vi "Main_spb.vi"() -> ()   [LabVIEW 2018]
uses:
  <vilib>/Platform/TimedLoop/XDataNode/timing_clust.ctl
  <vilib>/Platform/TimedLoop/XDataNode/nitl_modes.ctl
  <vilib>/Platform/TimedLoop/XDataNode/wakeup.ctl
  <vilib>/rvi/eio/common/nirviEmuTemplateMethod_errors.vi
  <vilib>/rvi/Emulation/niFpgaGetClockAttributes.vi
  <vilib>/rvi/Emulation/niFpgaSctlEmulationGetInTimedLoop.vi
  <vilib>/rvi/Emulation/niFpgaEmulationReportErrorSimple.vi
  <vilib>/rvi/Emulation/niFpgaProcessEmulError.vi
  <vilib>/rvi/Emulation/niFpgaCriticalErrorInLSC.vi
  <vilib>/rvi/DataTransferAndStorage/Container/Common/niFpgaContainerGetUniqueNameForEmu.vi
  <vilib>/rvi/Memory/Memory_Emulation/niFpgaMemoryFastEmulationDramWriteAndRequestData.vi
  <vilib>/rvi/Memory/Memory_Emulation/niFpgaMemoryEmulationDramWriteAndRequestData.vi
  <vilib>/rvi/Memory/Memory_Emulation/niFpgaMemoryEmulationDramWriteAndRequestDataApplyByteEnables.vi
  <vilib>/rvi/interface/RandomDataEmulation/niFpgaRandomDataHandleErrors.vi
  <vilib>/eio/EIONode/EIONode.xnode
  <vilib>/Platform/TimedLoop/XDataNode/XDataNode.xnode
  <vilib>/rvi/DataTransferAndStorage/Container/XNode/niFpgaContainer.xnode
  <vilib>/rvi/Memory/Memory_Emulation/niFpgaMemoryEmulationDramRetrieveData.vi
  <vilib>/rvi/interface/RandomDataEmulation/nirviRandomDataFpgaReadWriteTemplate.vi
  <vilib>/Platform/TimedLoop/XDataNode/XDNodeRunTimeDep.lvlib
panel:
  in  "RELAY_18_IN1":bool
  in  "RELAY_18_IN2":bool
  in  "RELAY_28_IN1":bool
  in  "RELAY_28_IN2":bool
  in  "RELAY_30_IN1":bool
  in  "RELAY_30_IN2":bool
  out "I":i32
  in  "Свет до":u32
  in  "Свет от":u32
  in  "Задержка":u32
  in  "Линейки":bool
  in  "Свет":bool
  in  "10":i8=10
  in  "30":i8=30
  in  "Кадр на ПК 16384":bool
  in  "Нач_адр":u32
  in  "2":u8=2
  in  "4":u8=4
  in  "Кон_адр":u32=16384
  out "Записали FIFO":bool
  in  "Строка триггер":u16=1200
  in  "Остановка основного цикла":bool
  in  "Горизонталы":i32=1048
  in  "H1_1":i8=10
  in  "H1_2":i8=36
  in  "H2_1":i8=3
  in  "H2_2":i8=28
  in  "H3_1":i8=20
  in  "H3_2":i8=45
  in  "RG_1":i8=6
  in  "RG_2":i8=16
  in  "48":i8=48
  in  "После H, мкс":u16=15
  in  "CDS1_1":i8=20
  in  "CDS1_2":i8=24
  in  "CDS2_1":i8=36
  in  "CDS2_2":i8=47
  in  "ADC_1":i8=20
  in  "ADC_2":i8=41
  in  "Задержка после переноса строки, мкс":u16=15
  in  "1800":i16=1800
  in  "S3_1":i16=50
  in  "S3_2":i16=950
  in  "S2_1":i16=600
  in  "S2_2":i16=1500
  in  "S1_1":i16=300
  in  "S1_2":i16=1200
  out "Сколько адресов записали?":u32
  in  "Сколько строк?":i32=2047
  in  "Read(T)/Write(F)":bool
  in  "Enum":T1(ring)
  in  "Write Data":bool[](array[boolean])=[FALSE, FALSE, FALSE, FALSE, FALSE, FALSE, FALSE, FALSE, FALSE]
  in  "8":i8=8
  out "READ":bool[](array[boolean])
  in  "18":i8=18
  in  "7":i8=7
  in  "18_1":i8=18
  in  "Конфигурация":bool
  in  "Кадр в память":bool
  in  "Command array":bool[](array[boolean])=[FALSE, FALSE, FALSE, FALSE, FALSE, FALSE, FALSE, FALSE, FALSE, FALSE, FALSE, FALSE, FALSE, FALSE, FALSE, FALSE, FALSE]
  # "Чтобы записать кадр в память,\nсначала \"Кадр в память\", затем\nкнопка \"Автомат\""
  # "8"
  # "0"
  # "8"
  # "0"
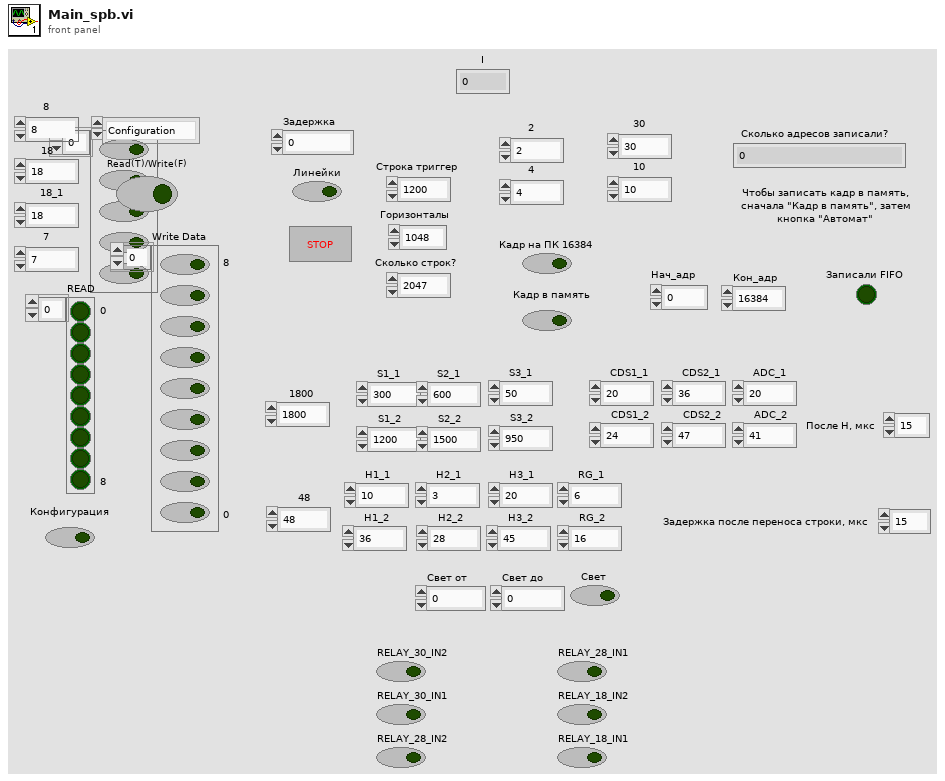
[diagram p1: front panel]
types:
  T1 = enum16{"Configuration", "MUX", "RED PGA", "GREEN PGA", "BLUE PGA", "RED OFF", "GREEN OFF", "BLUE OFF"}
  T2 = typedef "XDNodeRunTimeDep.lvlib/timing_clust.ctl" = cluster{"Expected End [f-1]":u64, "Actual End [f-1]":u64, "Finished Late? [f-1]":bool, "Expected End [i-1]":u64, "Actual End [i-1]":u64, "Finished Late? [i-1]":bool, "Expected Start [i]":u64, "Actual Start [i]":u64, "Expected Start [f]":u64, "Actual Start [f]":u64, "Source Name":string, "Structure Name":string, "Period":i64, "Deadline":i64, "Offset":i64, "Start":i64, "Priority":i32, "Timeout":i32, "Mode":T3, "Wakeup Reason":T4, "Error":errorcluster, "Source Type":string, "Secondary Source Type":string, "Global End Time":u64, "Global Start Time":u64, "Frame Duration":u64, "Iteration Duration":u64, "Assigned CPU":i32, "I/O Scan Engine Mode":u32}
  T3 = typedef "XDNodeRunTimeDep.lvlib/nitl_modes.ctl" = enum32{"No Change", "Process missed periods, maintain original phase", "Discard missed periods, maintain original phase", "Process missed periods, ignore original phase", "Discard missed periods, ignore original phase"}
  T4 = typedef "XDNodeRunTimeDep.lvlib/wakeup.ctl" = enum32{"Normal", "Aborted", "Asynchronous wakeup", "Timing source error", "Timed loop error", "Timeout"}
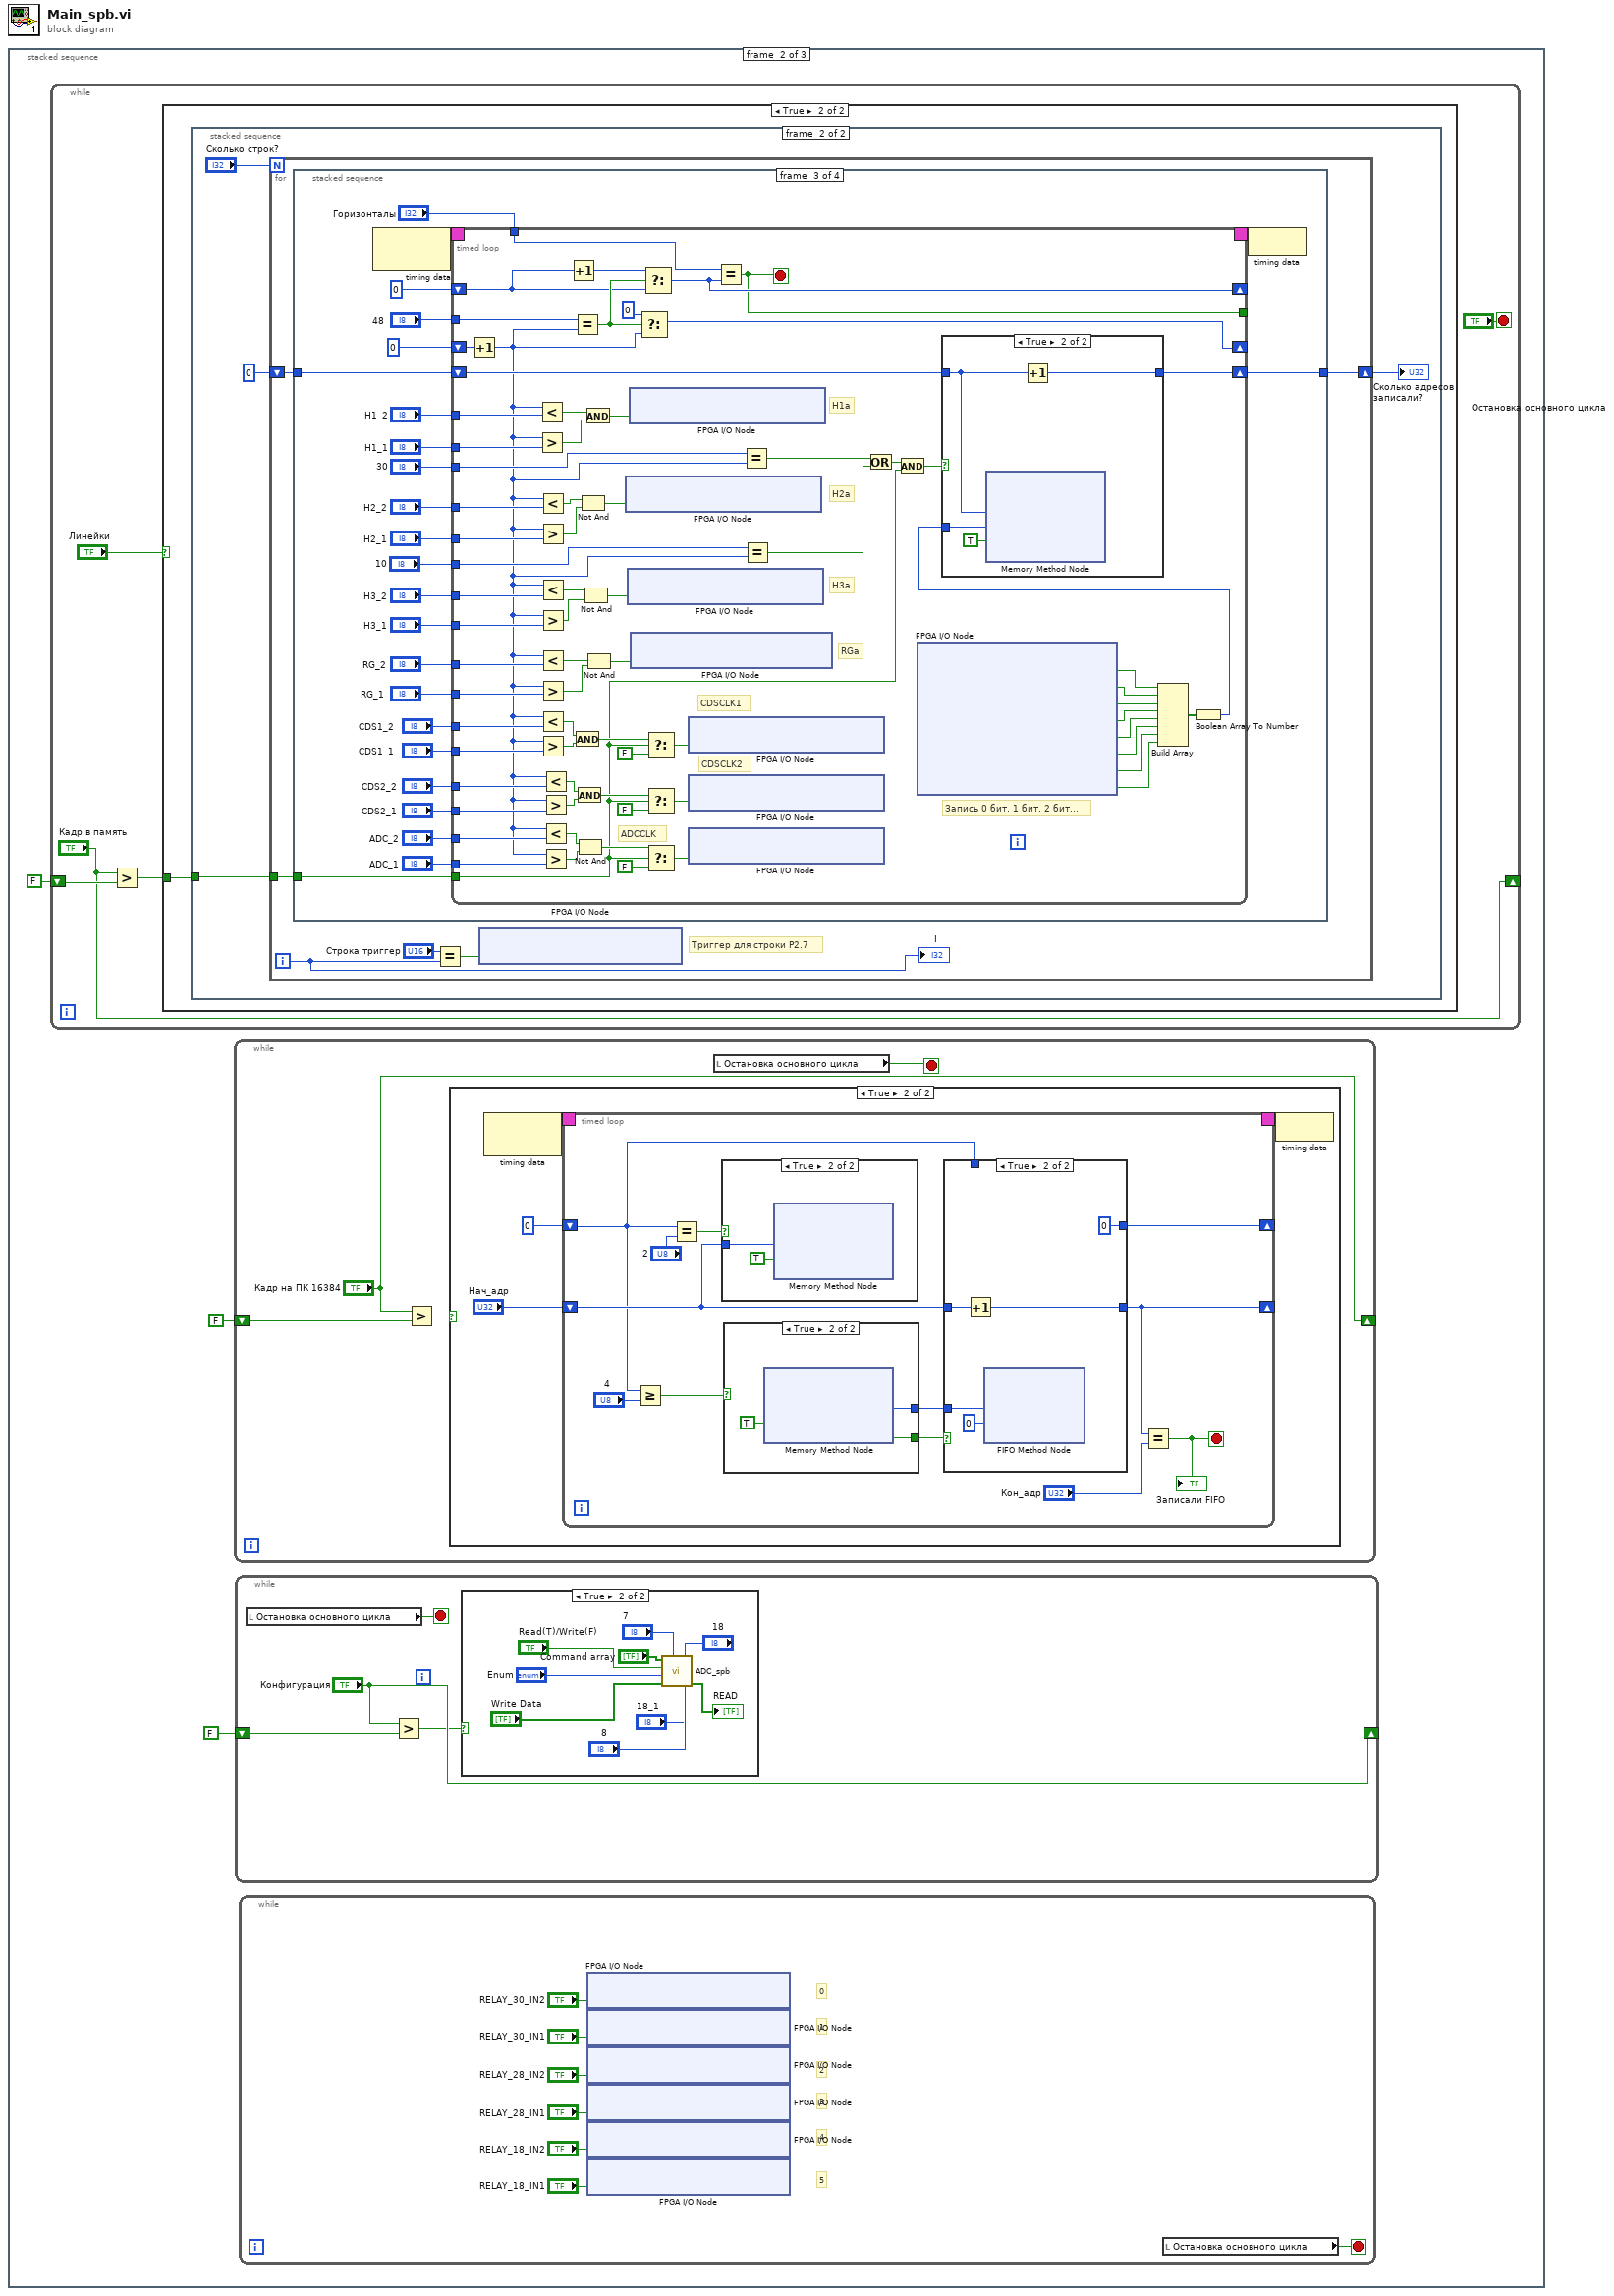
[diagram p0: block diagram]
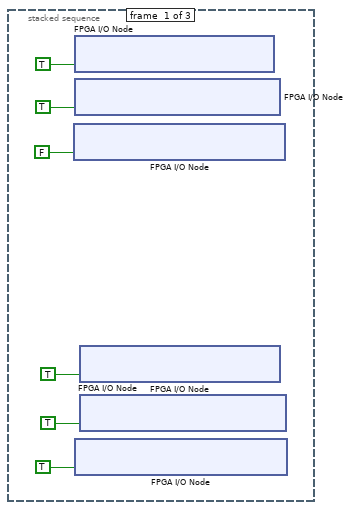
[diagram p2: hidden frame]
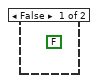
[diagram p3: hidden frame]
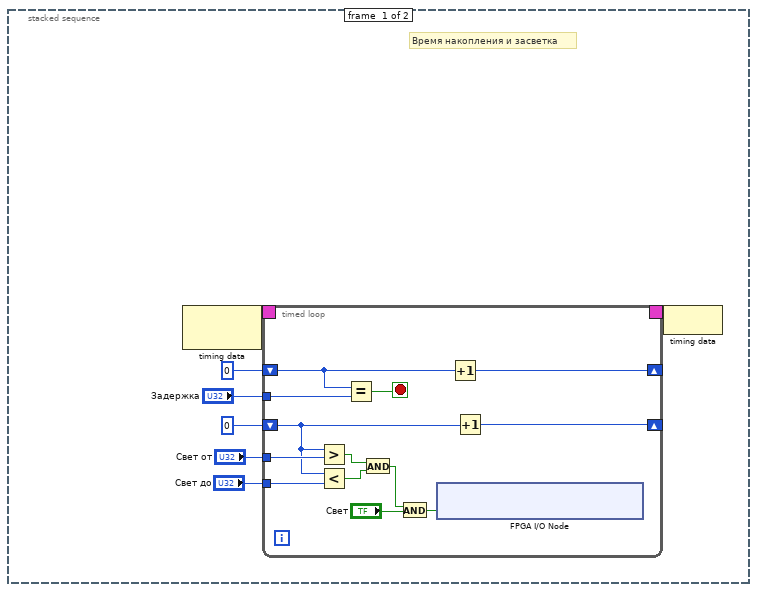
[diagram p4: hidden frame]
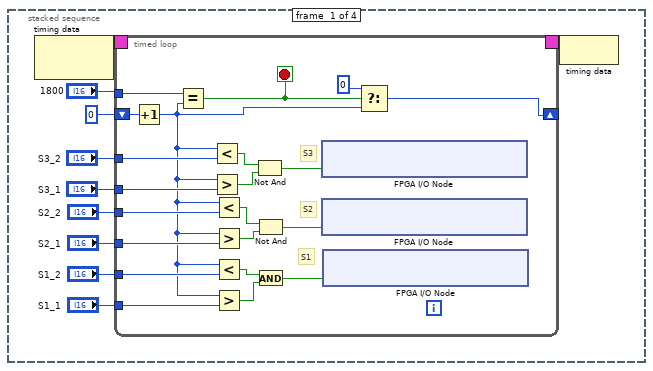
[diagram p5: hidden frame]
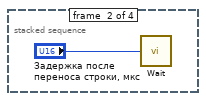
[diagram p6: hidden frame]
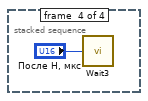
[diagram p8: hidden frame]
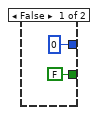
[diagram p10: hidden frame]
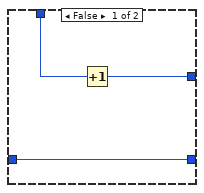
[diagram p12: hidden frame]
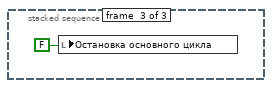
[diagram p14: hidden frame]
diagram:
  n1 = stacked-sequence {
    frame #0 {
      n2 = xnode "FPGA I/O Node"("IO Module\\DDCB_DIO16-23_WE"=FALSE ("IO Module\\DDCB_DIO16-23_WE")) -> ()  [unwired: 1 in, 1 out]
      n3 = xnode "FPGA I/O Node"("IO Module\\DDCB_DIO0-7_WE"=TRUE) -> ()  [unwired: 1 in, 1 out]
      n4 = xnode "FPGA I/O Node"("IO Module\\DDCB_DIO8-15_WE"=TRUE) -> ()  [unwired: 1 in, 1 out]
      n5 = xnode "FPGA I/O Node"("IO Module\\DDCA_DIO16-23_WE"=TRUE) -> ()  [unwired: 1 in, 1 out]
      n6 = xnode "FPGA I/O Node"("IO Module\\DDCA_DIO0-7_WE"=TRUE) -> ()  [unwired: 1 in, 1 out]
      n7 = xnode "FPGA I/O Node"("IO Module\\DDCA_DIO8-15_WE"=TRUE) -> ()  [unwired: 1 in, 1 out]
    }
    frame #1 {
      n8 = while {
        shift-right: ["Кадр в память"] -> _
        shift-left: FALSE ("Кадр в память") -> [w19]
        stop <- "Остановка основного цикла" stop-if-true
        n9 = Greater?(x="Кадр в память", y=w19) -> (0:w18:bool)
        n10 = case shown="True" "Линейки" {
          tunnel: w18 -> [_ w22]
          frame False {
            (unwired) FALSE ("Кадр в память")
          }
          frame True {
            n11 = stacked-sequence {
              tunnel: w22 -> [_ w47]
              frame #0 {
                # "Время накопления и засветка"
                n12 = node-c288() -> (w29:T2)  [unwired: 1 in]
                n13 = timed-loop {
                  timing: w29 -> [_]
                  timing-out: [_] -> w28
                  shift-right: [w39] -> _
                  shift-left: u32 0 -> [w40]
                  tunnel: "Задержка" -> [w42]
                  shift-right: [w33] -> _
                  shift-left: u32 0 -> [w34]
                  tunnel: "Свет от" -> [w38]
                  tunnel: "Свет до" -> [w37]
                  stop <- w41 stop-if-true
                  n14 = Greater?(x=w34, y=w38) -> (0:w36:bool)
                  n15 = Less?(x=w34, y=w37) -> (x < y?=w35:bool)
                  n16 = Equal?(x=w40, y=w42) -> (x = y?=w41:bool)
                  n17 = And(x=w36, y=w35) -> (x .and. y?=w31:bool)
                  n18 = And(x=w31, y="Свет") -> (x .and. y?=w32:bool)
                  n19 = xnode "FPGA I/O Node"("IO Module\\DDCA_DIO22_Write"=w32) -> ()  [unwired: 1 in, 1 out]
                  n20 = Increment(x=w40) -> (x+1=w39:u32)
                  n21 = Increment(x=w34) -> (x+1=w33:u32)
                }
                n22 = node-c288(w28) -> ()
              }
              frame #1 {
                n23 = for {
                  N: "Сколько строк?" -> [_]
                  shift-right: [w55] -> w48
                  shift-left: u32 0 -> [w56]
                  tunnel: w47 -> [w52]
                  i -> [w51]
                  # "Триггер для строки Р2.7"
                  n24 = stacked-sequence {
                    tunnel: w56 -> [_ _ w117 _]
                    tunnel: [_ _ w116 _] -> w55
                    tunnel: w52 -> [_ _ w93 _]
                    frame #0 {
                      n25 = node-c288() -> (w66:T2)  [unwired: 1 in]
                      n26 = timed-loop {
                        shift-right: [w85] -> _
                        shift-left: i16 0 -> [w87]
                        timing: w66 -> [_]
                        timing-out: [_] -> w65
                        tunnel: "1800" -> [w84]
                        tunnel: "S3_2" -> [w74]
                        tunnel: "S3_1" -> [w73]
                        tunnel: "S2_2" -> [w72]
                        tunnel: "S2_1" -> [w71]
                        tunnel: "S1_2" -> [w70]
                        tunnel: "S1_1" -> [w69]
                        stop <- w68 stop-if-true
                        # "S1"
                        # "S2"
                        # "S3"
                        n27 = Increment(x=w87) -> (x+1=w67:i16)
                        n28 = Equal?(x=w84, y=w67) -> (x = y?=w68:bool)
                        n29 = Less?(x=w67, y=w74) -> (x < y?=w78:bool)
                        n30 = Greater?(x=w67, y=w73) -> (0:w79:bool)
                        n31 = Less?(x=w67, y=w72) -> (x < y?=w80:bool)
                        n32 = Greater?(x=w67, y=w71) -> (0:w81:bool)
                        n33 = Less?(x=w67, y=w70) -> (x < y?=w82:bool)
                        n34 = Greater?(x=w67, y=w69) -> (0:w83:bool)
                        n35 = Not And(1:w79, 2:w78) -> (0:w77:bool)
                        n36 = Not And(1:w81, 2:w80) -> (0:w76:bool)
                        n37 = And(x=w82, y=w83) -> (x .and. y?=w75:bool)
                        n38 = xnode "FPGA I/O Node"("IO Module\\DDCB_DIO11_Write"=w77) -> ()  [unwired: 1 in, 1 out]
                        n39 = xnode "FPGA I/O Node"("IO Module\\DDCB_DIO12_Write"=w76) -> ()  [unwired: 1 in, 1 out]
                        n40 = xnode "FPGA I/O Node"("IO Module\\DDCB_DIO13_Write"=w75) -> ()  [unwired: 1 in, 1 out]
                        n41 = Select(t=i16 0, s=w68, f=w67) -> (s? t:f=w85:i16)
                      }
                      n42 = node-c288(w65) -> ()
                    }
                    frame #1 {
                      n43 = call "Wait"("Count(uSec)"="Задержка после переноса строки, мкс") -> ()  [unwired: 1 out]
                    }
                    frame #2 {
                      n44 = node-c288() -> (w115:T2)  [unwired: 1 in]
                      n45 = timed-loop {
                        timing: w115 -> [_]
                        timing-out: [_] -> w114
                        tunnel: "H1_2" -> [w184]
                        tunnel: "H1_1" -> [w183]
                        tunnel: "H2_2" -> [w188]
                        tunnel: "H2_1" -> [w187]
                        tunnel: "H3_2" -> [w186]
                        tunnel: "H3_1" -> [w185]
                        shift-right: [w177] -> _
                        shift-left: i8 0 -> [w182]
                        tunnel: "RG_2" -> [w181]
                        tunnel: "RG_1" -> [w180]
                        tunnel: "48" -> [w179]
                        tunnel: "Горизонталы" -> [w161]
                        shift-right: [w160] -> _
                        shift-left: 0 -> [w162]
                        tunnel: [w159] -> _
                        tunnel: "CDS1_2" -> [w152]
                        tunnel: "CDS1_1" -> [w151]
                        tunnel: "CDS2_2" -> [w150]
                        tunnel: "CDS2_1" -> [w149]
                        tunnel: "ADC_2" -> [w148]
                        tunnel: "ADC_1" -> [w147]
                        shift-right: [w126] -> w116
                        shift-left: w117 -> [w127]
                        tunnel: "30" -> [w121]
                        tunnel: "10" -> [w120]
                        tunnel: w93 -> [w118]
                        stop <- w159 stop-if-true
                        # "Запись 0 бит, 1 бит, 2 бит..."
                        # "ADCCLK"
                        # "CDSCLK2"
                        # "CDSCLK1"
                        # "H3a"
                        # "H2a"
                        # "H1a"
                        # "RGa"
                        n46 = Increment(x=w182) -> (x+1=w119:i8)
                        n47 = Less?(x=w119, y=w184) -> (x < y?=w176:bool)
                        n48 = Greater?(x=w119, y=w183) -> (0:w175:bool)
                        n49 = Less?(x=w119, y=w188) -> (x < y?=w174:bool)
                        n50 = Greater?(x=w119, y=w187) -> (0:w173:bool)
                        n51 = Less?(x=w119, y=w186) -> (x < y?=w172:bool)
                        n52 = Greater?(x=w119, y=w185) -> (0:w171:bool)
                        n53 = Less?(x=w119, y=w181) -> (x < y?=w170:bool)
                        n54 = Greater?(x=w119, y=w180) -> (0:w169:bool)
                        n55 = Less?(x=w119, y=w152) -> (x < y?=w153:bool)
                        n56 = Greater?(x=w119, y=w151) -> (0:w154:bool)
                        n57 = Less?(x=w119, y=w150) -> (x < y?=w156:bool)
                        n58 = Greater?(x=w119, y=w149) -> (0:w155:bool)
                        n59 = Less?(x=w119, y=w148) -> (x < y?=w157:bool)
                        n60 = Greater?(x=w119, y=w147) -> (0:w158:bool)
                        n61 = Increment(x=w162) -> (x+1=w163:i32)
                        n62 = Equal?(x=w179, y=w119) -> (x = y?=w164:bool)
                        n63 = And(x=w153, y=w154) -> (x .and. y?=w144:bool)
                        n64 = And(x=w156, y=w155) -> (x .and. y?=w143:bool)
                        n65 = Not And(1:w158, 2:w157) -> (0:w142:bool)
                        n66 = Not And(1:w173, 2:w174) -> (0:w166:bool)
                        n67 = Not And(1:w171, 2:w172) -> (0:w165:bool)
                        n68 = And(x=w176, y=w175) -> (x .and. y?=w167:bool)
                        n69 = Not And(1:w169, 2:w170) -> (0:w168:bool)
                        n70 = xnode "FPGA I/O Node"("IO Module\\DDCB_DIO5_Write"=w166) -> ()  [unwired: 1 in, 1 out]
                        n71 = xnode "FPGA I/O Node"("IO Module\\DDCB_DIO6_Write"=w165) -> ()  [unwired: 1 in, 1 out]
                        n72 = xnode "FPGA I/O Node"("IO Module\\DDCB_DIO4_Write"=w167) -> ()  [unwired: 1 in, 1 out]
                        n73 = xnode "FPGA I/O Node"("IO Module\\DDCB_DIO10_Write"=w168) -> ()  [unwired: 1 in, 1 out]
                        n74 = Select(t=i8 0, s=w164, f=w119) -> (s? t:f=w177:i8)
                        n75 = Select(t=w163, s=w164, f=w162) -> (s? t:f=w160:i32)
                        n76 = Select(t=w144, s=w118, f=FALSE) -> (s? t:f=w146:bool)
                        n77 = Select(t=w143, s=w118, f=FALSE) -> (s? t:f=w145:bool)
                        n78 = Select(t=w142, s=w118, f=FALSE) -> (s? t:f=w138:bool)
                        n79 = xnode "FPGA I/O Node"("IO Module\\DDCB_DIO0_Write"=w146) -> ()  [unwired: 1 in, 1 out]
                        n80 = xnode "FPGA I/O Node"("IO Module\\DDCB_DIO3_Write"=w145) -> ()  [unwired: 1 in, 1 out]
                        n81 = xnode "FPGA I/O Node"("IO Module\\DDCB_DIO1_Write"=w138) -> ()  [unwired: 1 in, 1 out]
                        n82 = Equal?(x=w161, y=w160) -> (x = y?=w159:bool)
                        n83 = Equal?(x=w121, y=w119) -> (x = y?=w123:bool)
                        n84 = Equal?(x=w120, y=w119) -> (x = y?=w122:bool)
                        n85 = Or(x=w123, y=w122) -> (x .or. y?=w125:bool)
                        n86 = And(x=w125, y=w118) -> (x .and. y?=w124:bool)
                        n87 = xnode "FPGA I/O Node"() -> ("IO Module\\DDCB_DIO16_Read"=w137:bool, "IO Module\\DDCB_DIO17_Read"=w136:bool, "IO Module\\DDCB_DIO18_Read"=w135:bool, "IO Module\\DDCB_DIO19_Read"=w134:bool, "IO Module\\DDCB_DIO20_Read"=w133:bool, "IO Module\\DDCB_DIO21_Read"=w132:bool, "IO Module\\DDCB_DIO22_Read"=w131:bool, "IO Module\\DDCB_DIO23_Read"=w130:bool)  [unwired: 8 in, 8 out]
                        n88 = Build Array(w137, w136, w135, w134, w133, w132, w131, w130) -> (w129:bool[])
                        n89 = Boolean Array To Number(Boolean array=w129) -> (number=w128:u8)
                        n90 = case shown="True" w124 {
                          tunnel: w128 -> [_ w192]
                          tunnel: w127 -> [w189 w190]
                          tunnel: [w189 w191] -> w126
                          frame False {
                          }
                          frame True {
                            n91 = xnode ("Memory Method Node")("Address"=w190, "Data"=w192, "Input Valid"=TRUE) -> ()  [unwired: 1 in, 2 out]
                            n92 = Increment(x=w190) -> (x+1=w191:u32)
                          }
                        }
                      }
                      n93 = node-c288(w114) -> ()
                    }
                    frame #3 {
                      n94 = call "Wait3"("Count(uSec)"="После H, мкс") -> ()  [unwired: 1 out]
                    }
                  }
                  n95 = Equal?(x="Строка триггер", y=w51) -> (x = y?=w53:bool)
                  n96 = xnode "FPGA I/O Node"("IO Module\\DDCA_DIO23_Write"=w53) -> ()  [unwired: 1 in, 1 out]
                  "I" <- w51
                }
                "Сколько адресов записали?" <- w48
              }
            }
          }
        }
      }
      n97 = while {
        shift-right: ["Кадр на ПК 16384"] -> _
        shift-left: FALSE ("Кадр на ПК поадресно") -> [w201]
        stop <- w202 stop-if-true
        n98 = Greater?(x="Кадр на ПК 16384", y=w201) -> (0:w199:bool)
        n99 = case shown="True" w199 {
          frame False {
          }
          frame True {
            n100 = node-c288() -> (w206:T2)  [unwired: 1 in]
            n101 = timed-loop {
              shift-right: [w217] -> _
              shift-left: "Нач_адр" -> [w211]
              timing: w206 -> [_]
              timing-out: [_] -> w205
              shift-right: [w208] -> _
              shift-left: u8 0 -> [w209]
              stop <- w218 stop-if-true
              n102 = Greater Or Equal?(x=w209, y="4") -> (x >= y?=w212:bool)
              n103 = Equal?(x=w209, y="2") -> (x = y?=w215:bool)
              n104 = case shown="True" w215 {
                tunnel: w211 -> [_ w224]
                frame False {
                }
                frame True {
                  n105 = xnode ("Memory Method Node")("Address"=w224, "Input Valid"=TRUE) -> ()  [unwired: 1 in, 2 out]
                }
              }
              n106 = case shown="True" w212 {
                tunnel: [u8 0 ("Data") w222] -> w216
                tunnel: [FALSE ("Output Valid") w221] -> w210
                frame False {
                }
                frame True {
                  n107 = xnode ("Memory Method Node")("Ready for Output"=TRUE ("Ready For Output")) -> ("Data"=w222:u8, "Output Valid"=w221:bool)  [unwired: 1 in, 1 out]
                }
              }
              n108 = case shown="True" w210 {
                tunnel: [w226 w233] -> w217
                tunnel: w216 -> [_ w231]
                tunnel: w211 -> [w226 w230]
                tunnel: w209 -> [w228 _]
                tunnel: [w227 u8 0] -> w208
                frame False {
                  n109 = Increment(x=w228) -> (x+1=w227:u8)
                }
                frame True {
                  n110 = Increment(x=w230) -> (x+1=w233:u32)
                  n111 = xnode ("FIFO Method Node")("Element"=w231, "Timeout"=0) -> ()  [unwired: 1 in, 2 out]
                }
              }
              n112 = Equal?(x=w217, y="Кон_адр") -> (x = y?=w218:bool)
              "Записали FIFO" <- w218
            }
            n113 = node-c288(w205) -> ()
          }
        }
        n114 = local read "Остановка основного цикла"() -> (w202:bool)
      }
      n115 = while {
        shift-right: ["Конфигурация"] -> _
        shift-left: FALSE ("Конфигурация") -> [w240]
        stop <- w241 stop-if-true
        n116 = local read "Остановка основного цикла"() -> (w241:bool)
        n117 = Greater?(x="Конфигурация", y=w240) -> (0:w238:bool)
        n118 = case shown="True" w238 {
          frame False {
          }
          frame True {
            n119 = call "ADC_spb.vi"(1:"18_1"="18", 2:"18_1"="18_1", "8"="8", "7"="7", "Write Data"="Write Data", "Enum"="Enum", "Read(T)/Write(F)"="Read(T)/Write(F)", "Command array"="Command array") -> ("READ"=→"READ":bool[])
          }
        }
      }
      n120 = while {
        stop <- w16 stop-if-true
        # "5"
        # "4"
        # "3"
        # "2"
        # "1"
        # "0"
        n121 = xnode "FPGA I/O Node"("IO Module\\DDCA_DIO16_Write"="RELAY_30_IN2") -> ()  [unwired: 1 in, 1 out]
        n122 = xnode "FPGA I/O Node"("IO Module\\DDCA_DIO17_Write"="RELAY_30_IN1") -> ()  [unwired: 1 in, 1 out]
        n123 = xnode "FPGA I/O Node"("IO Module\\DDCA_DIO18_Write"="RELAY_28_IN2") -> ()  [unwired: 1 in, 1 out]
        n124 = xnode "FPGA I/O Node"("IO Module\\DDCA_DIO19_Write"="RELAY_28_IN1") -> ()  [unwired: 1 in, 1 out]
        n125 = xnode "FPGA I/O Node"("IO Module\\DDCA_DIO20_Write"="RELAY_18_IN2") -> ()  [unwired: 1 in, 1 out]
        n126 = xnode "FPGA I/O Node"("IO Module\\DDCA_DIO21_Write"="RELAY_18_IN1") -> ()  [unwired: 1 in, 1 out]
        n127 = local read "Остановка основного цикла"() -> (w16:bool)
      }
    }
    frame #2 {
      n128 = local write "Остановка основного цикла"(FALSE) -> ()
    }
  }
